vi "Send message to TCP Server.vi"(7 "LabVIEW Object":refnum<class>, 8 "error in (no error)":errorcluster, 10 "String":string, 11 "Guardian ID":string) -> (0 "error out":errorcluster)   [LabVIEW 2026, in "TALOS.lvlib"]
uses:
  TALOS.lvlib
  Ancestor/Ancestor/Ancestor.lvclass/Ancestor.ctl
  Generate Error.vi
  Circus Config Param - Core.vi
  FGV/Error Memory/Get Error Description.vi
  Get PC name.vi
  Ancestor/Ancestor/Read ID.vi
  Get Class Name.vi
  <vilib>/Utility/error.llb/Clear Errors.vi
  Circus Root Path.vi
  TALOS Config Param.vi
  FGV/Error Memory/Error Memory Core.vi
  <vilib>/AdvancedString/Delimited String to 1D String Array.vi
  <vilib>/AdvancedString/Delimited String to 1D String Array (string).vi
  FGV/Error Memory/Error Crt Lvl checker.vi
  FGV/Error Memory/Error Memory Core.vi/40c8088d-b597-4017-91af-faa98e00292e.vi
  FGV/Error Memory/Error Memory Core.vi/d4a3ab98-063c-4e44-b43d-fbdcfe6c2be2.vi
  Global Constants.vi
  Global Memory.vi
  <vilib>/Utility/LVClass/Get LV Class Name.vi
  Is in Packed Library.vi
  TALOS Root path.vi
  Read CSV worksheet.vi
  <vilib>/Utility/error.llb/General Error Handler.vi
  <vilib>/Utility/config.llb/Open Config Data.vi
  <vilib>/Utility/config.llb/Get Section Names.vi
  <vilib>/Utility/config.llb/Get Key Names.vi
  <vilib>/Utility/config.llb/Read Key.vi
  <vilib>/Utility/config.llb/Read Key (String).vi
  <vilib>/Utility/config.llb/Close Config Data.vi
  Guardian/Guardian/Extract list from Project INI file entry.vi
  Error Log.vi
  Ancestor/Ancestor/Ancestor.lvclass
  <vilib>/Comparison/Equal/Equal Functor/Equal Functor.lvclass
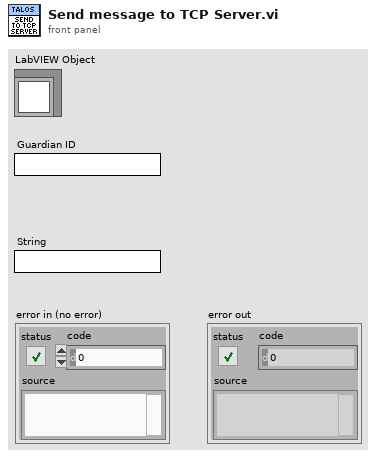
[diagram p1: front panel]
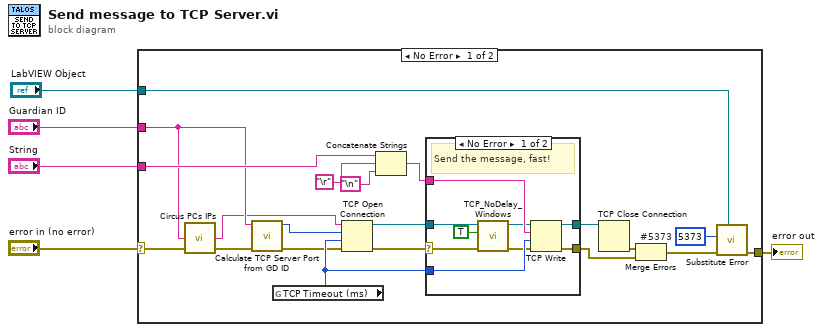
[diagram p0: block diagram]
diagram:
  n1 = case shown="No Error" "error in (no error)" {
    selector: "error in (no error)" -> [w11 w37]
    tunnel: "String" -> [w24 _]
    tunnel: "Guardian ID" -> [w7 _]
    tunnel: [w14 w37] -> w2
    tunnel: "LabVIEW Object" -> [w13 _]
    frame No Error {
      w16 = 5373  # #5373
      n2 = call "Circus PCs IPs.vi"("error in (no error)"=w11, "ID"=w7) -> ("error out"=w10:errorcluster, "IP"=w6:string)  [unwired: 2 in]
      n3 = call "Calculate TCP Server Port from GD ID.vi"("error in (no error)"=w10, "GD ID"=w7) -> ("error out"=w9:errorcluster, "Port"=w8:u16)  [unwired: 8 in]
      n4 = global read "Global Constants.vi" "TCP Timeout (ms)"() -> (w12:i32)
      n5 = TCP Open Connection(address=w6, remote port or service name=w8, timeout ms (60000)=w12, error in (no error)=w9) -> (connection ID=w20:refnum<k5>, error out=w19:errorcluster)  [unwired: 1 in]
      n6 = Concatenate Strings(w24, "\r", "\n") -> (w25:string)
      n7 = case shown="No Error" w19 {
        selector: w19 -> [w31 w35]
        tunnel: w12 -> [w34 _]
        tunnel: w25 -> [w33 _]
        tunnel: [w32 w36] -> w18
        tunnel: w20 -> [w28 w36]
        tunnel: [w26 w35] -> w21
        frame No Error {
          # "Send the message, fast!"
          n8 = call "TCP_NoDelay_Windows.vi"("error in (no error)"=w31, "TCP_NODELAY (true)"=TRUE, "connID"=w28) -> ("error out"=w30:errorcluster, "connID 2"=w29:refnum<k5>)  [unwired: 3 in]
          n9 = TCP Write(connection ID=w29, data in=w33, error in (no error)=w30, 9:w34) -> (connection ID out=w32:refnum<k5>, error out=w26:errorcluster)  [unwired: 1 out]
        }
        frame Error {
          # "Go straight to Close"
        }
      }
      n10 = TCP Close Connection(connection ID=w18) -> (error out=w17:errorcluster)  [unwired: 2 in, 1 out]
      n11 = Merge Errors(w17, w21) -> (w15:errorcluster)
      n12 = call "Substitute Error.vi"("LabVIEW Object"=w13, "error in (no error)"=w15, "Error Code"=w16) -> ("error out"=w14:errorcluster)  [unwired: 8 in]
    }
    frame Error {
    }
  }
  "error out" <- w2
